vi "Read Pin Map.vi"(8 "error in (no error)":errorcluster, 11 "NI-DAQ in":refnum<class "NI-DAQ.lvclass">) -> (0 "error out":errorcluster, 2 "Pin Map":T1={"Region Valves"=[49, 52, 0, 0], "Extra Valves"=[[[0.0, 48.0, 0.0, 0.0, 0.0]]], "Tool Primary Valve"=51, "Tool Secondary Valve"=50, "Region Sensors"=[37, 41, 37], "Extra Sensors"=[[[36.0, 37.0, 0.0, 0.0]]], "Tool Primary Sensor"=39.0, "Tool Secondary Sensor"=38.0, "Compression Sensor"=31.0, "5V"=50, "Dispenser Sensor"=0.0}, 3 "NI-DAQ out":refnum<class "NI-DAQ.lvclass">)   [LabVIEW 2021, in "NI-DAQ.lvclass"]
uses:
  NI-DAQ.lvclass
  Pin Map.ctl
  I-O.lvclass
panel:
  out "extra valves":i32[][][](array[numeric])
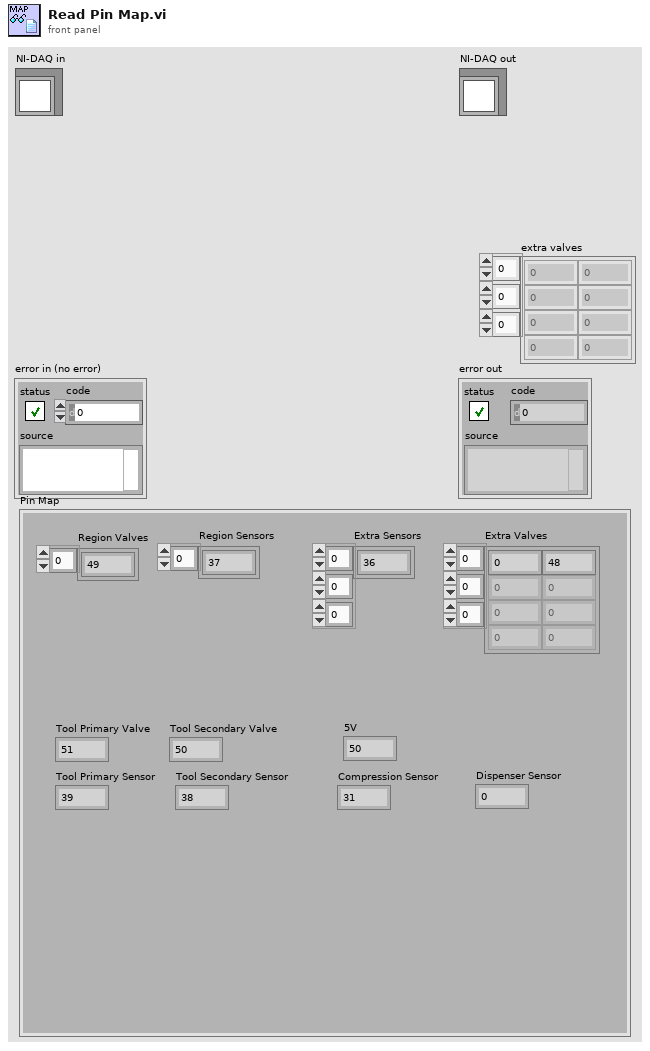
[diagram p1: front panel]
types:
  T1 = typedef "I-O.lvclass/Pin Map.ctl" = cluster{"Region Valves":i32[], "Extra Valves":dbl[][][], "Tool Primary Valve":i32, "Tool Secondary Valve":i32, "Region Sensors":i32[], "Extra Sensors":dbl[][][], "Tool Primary Sensor":dbl, "Tool Secondary Sensor":dbl, "Compression Sensor":dbl, "5V":i32, "Dispenser Sensor":dbl}
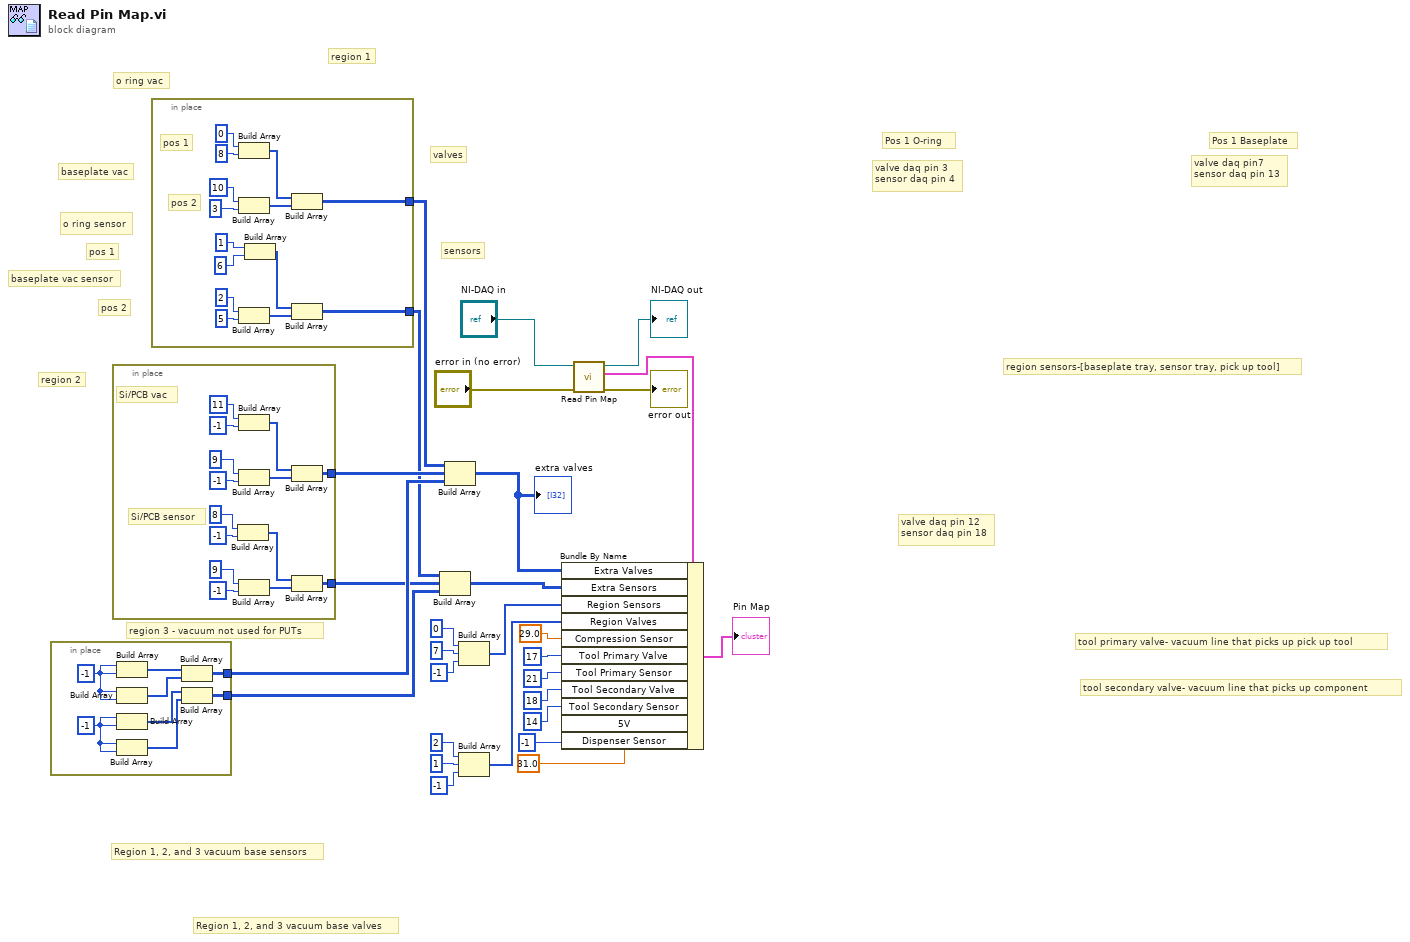
[diagram p0: block diagram]
diagram:
  # "o ring sensor"
  # "baseplate vac sensor"
  # "pos 2"
  # "pos 1"
  # "tool secondary valve- vacuum line that picks up component"
  # "tool primary valve- vacuum line that picks up pick up tool"
  # "valve daq pin 12\nsensor daq pin 18"
  # "Pos 1 Baseplate"
  # "Pos 1 O-ring"
  # "valve daq pin7 \nsensor daq pin 13"
  # "valve daq pin 3\nsensor daq pin 4"
  # "o ring vac"
  # "baseplate vac"
  # "region sensors-[baseplate tray, sensor tray, pick up tool]"
  # "region 3 - vacuum not used for PUTs"
  # "Region 1, 2, and 3 vacuum base sensors"
  # "Region 1, 2, and 3 vacuum base valves"
  # "region 2"
  # "sensors"
  # "valves"
  # "region 1"
  n1 = in-place {
    in-place-border: [w34] -> w8
    in-place-border: [w31] -> w5
    w30 = -1
    w36 = -1
    n2 = Build Array(w36, w36) -> (w37:i32[])
    n3 = Build Array(w36, w36) -> (w35:i32[])
    n4 = Build Array(w30, w30) -> (w33:i32[])
    n5 = Build Array(w30, w30) -> (w32:i32[])
    n6 = Build Array(w37, w35) -> (w34:i32[][])
    n7 = Build Array(w33, w32) -> (w31:i32[][])
  }
  n8 = in-place {
    in-place-border: [w45] -> w9
    in-place-border: [w38] -> w6
    # "Si/PCB sensor"
    # "Si/PCB vac"
    n9 = Build Array(8, -1) -> (w40:i32[])
    n10 = Build Array(11, -1) -> (w47:i32[])
    n11 = Build Array(9, -1) -> (w46:i32[])
    n12 = Build Array(9, -1) -> (w39:i32[])
    n13 = Build Array(w47, w46) -> (w45:i32[][])
    n14 = Build Array(w40, w39) -> (w38:i32[][])
  }
  n15 = in-place {
    in-place-border: [w59] -> w10
    in-place-border: [w52] -> w7
    # "pos 2"
    # "pos 1"
    n16 = Build Array(0, 8) -> (w60:i32[])
    n17 = Build Array "Build Array"(10, 3) -> (w61:i32[])
    n18 = Build Array(2, 5) -> (w54:i32[])
    n19 = Build Array(1, 6) -> (w53:i32[])
    n20 = Build Array(w60, w61) -> (w59:i32[][])
    n21 = Build Array(w53, w54) -> (w52:i32[][])
  }
  n22 = Build Array(w7, w6, w5) -> (w3:i32[][][])
  n23 = Build Array(w10, w9, w8) -> (w4:i32[][][])
  "extra valves" <- w4
  n24 = Build Array(0, 7, -1) -> (w11:i32[])
  n25 = Build Array(2, 1, -1) -> (w17:i32[])
  n26 = call-parent "Read Pin Map.vi"("error in (no error)"="error in (no error)", "I-O in"="NI-DAQ in") -> ("error out"=→"error out":errorcluster, "Pin Map 2"=w25:T1, "I-O out"=→"NI-DAQ out":refnum<class "NI-DAQ.lvclass">)  [unwired: 7 in]
  n27 = Bundle By Name(cluster=w25, "Extra Valves"=w4, "Extra Sensors"=w3, "Region Sensors"=w11, "Region Valves"=w17, "Compression Sensor"=29.0, "Tool Primary Valve"=17, "Tool Primary Sensor"=21 ("Tool Primary Valve"), "Tool Secondary Valve"=18 ("Tool Primary Valve"), "Tool Secondary Sensor"=14 ("Tool Secondary Valve"), "5V"=-1, "Dispenser Sensor"=31.0) -> (→"Pin Map":T1)
